vi "Initialize FPGA FIFOs.vi"(8 "error in (no error)":errorcluster, 11 "FGPA Ref":T1) -> (0 "error out":errorcluster, 3 "FGPA Ref":T1)   [LabVIEW 2013]
uses:
  RIG-SPECIFIC FILES/FPGA Refs/FPGA Ref.ctl
  <vilib>/rvi/interface/common/niFpgaWaitOnOcc.vi
  <vilib>/Utility/error.llb/Error Cluster From Error Code.vi
  <vilib>/rvi/interface/nirviMethod/nirviMethod.xnode
  <vilib>/rvi/errors/niLvFpgaMergeErrorWithErrorCode.vi
  <vilib>/FPGAPlugInAG/Dynamic/niLvFpga_StopFifo_Dynamic.vi
  <vilib>/FPGAPlugInAG/Dynamic/niLvFpga_StartFifo_Dynamic.vi
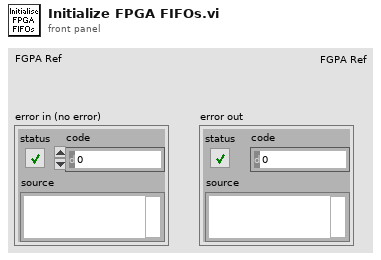
[diagram p1: front panel]
types:
  T1 = typedef "FPGA Ref.ctl" = refnum<k20>
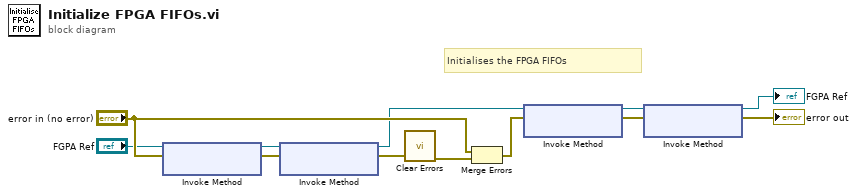
[diagram p0: block diagram]
diagram:
  # "Initialises the FPGA FIFOs"
  n1 = xnode ("Invoke Method")("FPGA VI Reference In"="FGPA Ref", "error in"="error in (no error)") -> ("FPGA VI Reference Out"=w9:T1, "error out"=w6:errorcluster)
  n2 = xnode "Invoke Method"("FPGA VI Reference In"=w9, "error in"=w6) -> ("FPGA VI Reference Out"=w2:T1, "error out"=w5:errorcluster)
  n3 = call <vilib>:"Clear Errors.vi"("error in (no error)"=w5) -> ("error out"=w7:errorcluster)  [unwired: 6 in]
  n4 = Merge Errors("error in (no error)", w7) -> (w11:errorcluster)
  n5 = xnode ("Invoke Method")("FPGA VI Reference In"=w2, "error in"=w11) -> ("FPGA VI Reference Out"=w12:T1, "error out"=w4:errorcluster)
  n6 = xnode "Invoke Method"("FPGA VI Reference In"=w12, "error in"=w4) -> ("FPGA VI Reference Out"=→"FGPA Ref":T1, "error out"=→"error out":errorcluster)
